vi "Example CPU Usage LV821.vi"() -> ()   [LabVIEW 2018]
doc: "This is the test VI from Donovan_B (https://forums.ni.com/t5/Example-Program-Drafts/Monitoring-CPU-usage-on-Windows-from-LabVIEW/ta-p/3520319?profile.language=en)"
panel:
  out "error out":errorcluster
  out "Processor History":sgl(graph)
  out "CPU Usage (%)":sgl(slide) scale=0.0..100.0
  in  "stop":bool
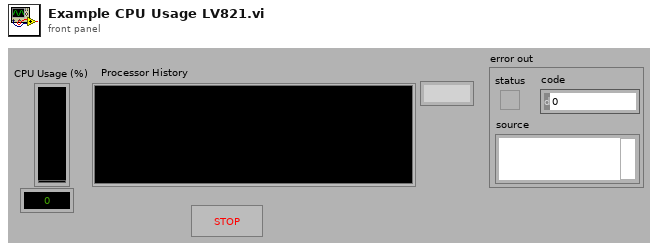
[diagram p1: front panel]
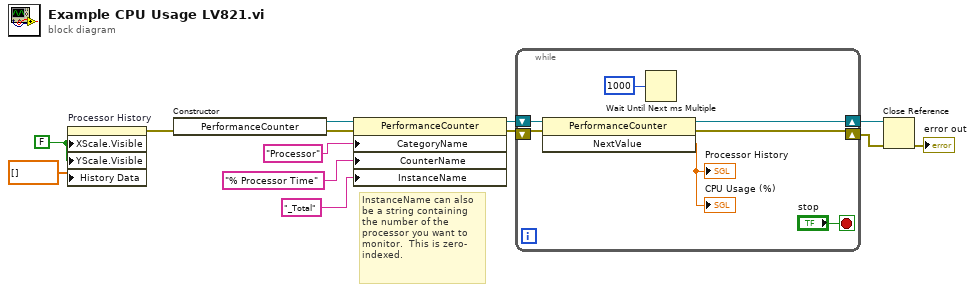
[diagram p0: block diagram]
diagram:
  w4 = FALSE ("X Scale.Visible")
  # "InstanceName can also\nbe a string containing\nthe number of the\nprocessor you want to\nmonitor.  This is zero-\nindexed."
  n1 = property on="Processor History" class="WFChart (strict)"("XScale.Visible"=w4, "YScale.Visible"=w4, "History Data"=sgl[] []) -> (error out=w1:errorcluster)  [unwired: 2 in, 1 out]
  n2 = constructor class="PerformanceCounter" ("Constructor Node")(error in=w1) -> (reference out=w13:refnum<k24>, error out=w12:errorcluster)  [unwired: 2 in, 1 out]
  n3 = property on="Property Node" class="PerformanceCounter"(reference=w13, error in=w12, "CategoryName"="Processor", "CounterName"="% Processor Time", "InstanceName"="_Total") -> (reference out=w9:refnum<k24>, error out=w8:errorcluster)
  n4 = while {
    shift-right: [w17] -> w6
    shift-left: w9 -> [w20]
    shift-right: [w18] -> w7
    shift-left: w8 -> [w19]
    stop <- "stop" stop-if-true
    n5 = invoke on="Invoke Node" class="PerformanceCounter" method="NextValue"(reference=w20, error in=w19) -> (reference out=w17:refnum<k24>, error out=w18:errorcluster, "NextValue"=→"CPU Usage (%)" →"Processor History":sgl)  [unwired: 1 in]
    n6 = Wait Until Next ms Multiple(millisecond multiple=u32 1000 ("milliseconds to wait")) -> ()  [unwired: 1 out]
  }
  n7 = Close Reference(reference=w6, error in (no error)=w7) -> (error out=→"error out":errorcluster)
